vi "SelectBeads.vi"(11 "Input image":T1) -> ()   [LabVIEW 2011]
uses:
  <vilib>/vision/Image Controls.llb/IMAQ Image.ctl
  GlobalVariables.vi
panel:
  in  "Use old?":bool
  in  "error in (no error)":errorcluster
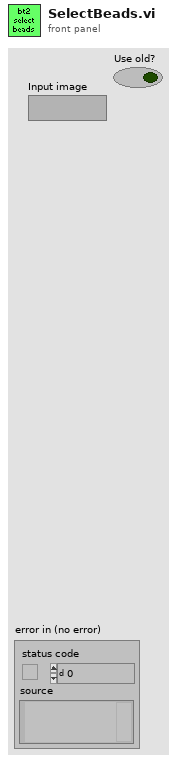
[diagram p1: front panel]
types:
  T1 = typedef "IMAQ Image.ctl" = refnum<image>
  T2 = typedef "MeasureConfigType.ctl" = cluster{"Bead locations":cluster{"X":i32, "Y":i32}[], "ROI":i32, "Experiment base path":path, "Image output subdir":string, "Output mode":T3, "Traces output subdir":string, "QTrk Settings":T4, "Tracking Config":T5, "Experiment Name":string, "Program":T8, "ZLUT":sgl[][][], "Camera settings":T15, "Experiment Script":string, "Max frames in memory":i32, "Save traces as binary":bool, "Pixel Calibration Gain Image":string, "Pixel Calibration Offset Image":string, "Use pixel calibration images":bool, "Internal camera settings":string}
  T3 = typedef "MeasureConfigOutputMode.ctl" = enum16{"None", "Track", "SaveImages"}
  T4 = typedef "QTrkSettings.ctl" = cluster{"Image width":i32, "Image height":i32, "Number of threads (CPU based)":i32, "CUDA Device":i32, "COM Background correction factor":sgl, "ZLUT MinRadius":sgl, "ZLUT Radial sample density":sgl, "ZLUT Angular sample density":sgl, "ZLUT ROI Coverage":sgl, "QI Iterations":i32, "QI MinRadius":sgl, "QI Radial sample density":sgl, "QI Angular sample density":sgl, "QI ROI Coverage":sgl, "QI Angular Step \nIteration Factor":sgl, "XCOR Profile Length":i32, "XCOR Profile Width":i32, "XCOR Iterations":i32, "Gaussian 2D Fit Iterations":i32, "Gaussian 2D Sigma (pixels)":sgl}
  T5 = typedef "TrackingConfigType.ctl" = cluster{"Number of steps":i32, "ZLUT stepsize (um)":sgl, "Z correction factor":sgl, "Start piezo Z (um)":sgl, "Pixel size (nm)":sgl, "2D Localization Type":T6, "Z Command (None)":T7, "Z Piezo scale":bool}
  T6 = typedef "QTrkLocalizationType.ctl" = enum16{"Center-of-Mass", "1D Cross-Correlation", "Quadrant Interpolation", "Gaussian 2D MLE", "QI + ZLUTAlign", "ZLUTAlign"}
  T7 = typedef "QTrkZCommandType.ctl" = enum16{"Nothing", "ComputeZ", "BuildRadialZLUT", "BuildImageZLUT", "RadialZLUT+ImageZLUT"}
  T8 = typedef "ExperimentProgramType.ctl" = cluster{"Commands":T9[], "Motor Axis accuracy conditions":T12, "Axis flags":T14}
  T9 = typedef "ExProgCommandType.ctl" = cluster{"cmd":T10, "axis":T11, "value/pos":dbl, "speed":dbl, "name":string}
  T10 = typedef "ExProgCommandEnumType.ctl" = enum16{"wait", "move", "acquire", "idle", "rmove", "when", "section", "stop"}
  T11 = typedef "MotorAxisEnum.ctl" = enum16{"no axis", "magrot", "magpos", "px", "py", "pz", "camx", "camy"}
  T12 = typedef "MotorPosType.ctl" = cluster{"Magnet Z":dbl, "Magnet rotation":dbl, "Camera":T13, "Piezo XY":T13, "Piezo Z":dbl}
  T13 = typedef "XYf.ctl" = cluster{"X":sgl, "Y":sgl}
  T14 = typedef "MotorPosFlagsType.ctl" = cluster{"Magnet Z":bool, "Magnet rotation":bool, "Camera":cluster{"X":bool, "Y":bool}, "Piezo XY":cluster{"X":bool, "Y":bool}, "Piezo Z":bool}
  T15 = typedef "GenericCameraConfigType.ctl" = cluster{"Framerate (Hz)":i32, "Exposure time (us)":i32, "Image size":cluster{"Width":i32, "Height":i32}, "Number of buffers":i32}
  T16 = typedef "CameraInstance.ctl" = cluster{"VI refs":T17, "Camera state":variant}
  T17 = typedef "CameraInterface.ctl" = cluster{"Close":T18, "Get/Set generic config":T19, "Grab":T20, "Show Settings Dialog":T21, "AdjustBeadPos":T22, "Save/load camera settings":T23}
  T18 = typedef "CICloseType.ctl" = refnum<vi>
  T19 = typedef "CIGetSetGenericConfig.ctl" = refnum<vi>
  T20 = typedef "CIGrabType.ctl" = refnum<vi>
  T21 = typedef "CISettingsDlg.ctl" = refnum<vi>
  T22 = typedef "CIAdjustBeadPos.ctl" = refnum<vi>
  T23 = typedef "CISaveLoadSettings.ctl" = refnum<vi>
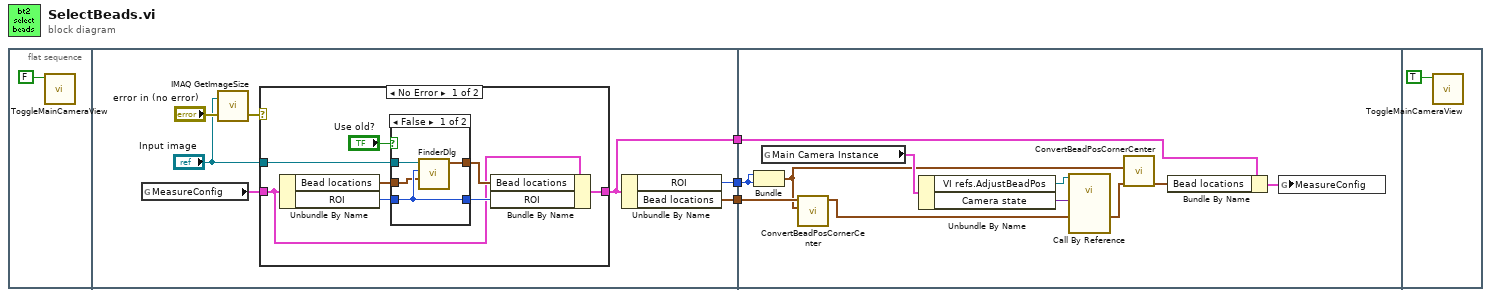
[diagram p0: block diagram]
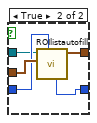
[diagram p2: hidden frame]
diagram:
  n1 = flat-sequence {
    tunnel: [w7] -> w3
    tunnel: [w6] -> w2
    tunnel: [w5] -> w1
    tunnel: w3 -> [w35]
    tunnel: w2 -> [w38]
    tunnel: w1 -> [w34]
    frame #0 {
      n2 = call "ToggleMainCameraView.vi"("Enable? (T)"=FALSE) -> ()  [unwired: 11 in]
    }
    frame #1 {
      n3 = global read "GlobalVariables.vi" "MeasureConfig"() -> (w8:T2)
      n4 = call "IMAQ GetImageSize"("Image"="Input image", "error in (no error)"="error in (no error)") -> ("error out"=w11:errorcluster)  [unwired: 2 in, 2 out]
      n5 = case shown="No Error" w11 {
        tunnel: "Input image" -> [w15 _]
        tunnel: w8 -> [w14 w29]
        tunnel: [w13 w29] -> w6
        frame No Error {
          n6 = Unbundle By Name(w14) -> ("Bead locations"=w19:cluster{"X":i32, "Y":i32}[], "ROI"=w18:i32)
          n7 = case shown="False" "Use old?" {
            tunnel: w19 -> [w20 w28]
            tunnel: w18 -> [w22 w27]
            tunnel: [w21 w26] -> w17
            tunnel: [w22 w25] -> w16
            tunnel: w15 -> [w23 w24]
            frame False {
              n8 = call "FinderDlg.vi"("Bead positions"=w20, "roi"=w22, "Input Image"=w23) -> ("Bead positions"=w21:cluster{"X":i32, "Y":i32}[])  [unwired: 8 in]
            }
            frame True {
              n9 = call "ROIlistautofill.vi"("ROI in (pix)"=w27, "Bead locations"=w28, "Image In"=w24) -> ("Output bead locations"=w26:cluster{"X":i32, "Y":i32}[], "ROI out"=w25:i32)  [unwired: 4 in, 3 out]
            }
          }
          n10 = Bundle By Name(cluster=w14, "Bead locations"=w17, "ROI"=w16) -> (w13:T2)
        }
        frame Error {
        }
      }
      n11 = Unbundle By Name(w6) -> ("ROI"=w5:i32, "Bead locations"=w7:cluster{"X":i32, "Y":i32}[])
    }
    frame #2 {
      n12 = Bundle("ROI"=w34, "ROI"=w34) -> (w32:cluster{"ROI":i32, "ROI":i32})  [unwired: 1 in]
      n13 = global read "GlobalVariables.vi" "Main Camera Instance"() -> (w36:T16)
      n14 = call "ConvertBeadPosCornerCenter.vi"("ROI Size"=w32, "Center-based bead locations"=w35) -> ("Corner-based bead pos (out)"=w33:cluster{"X":i32, "Y":i32}[])  [unwired: 8 in, 1 out]
      n15 = Unbundle By Name(w36) -> ("VI refs.AdjustBeadPos"=w39:T22, "Camera state"=w40:variant)
      n16 = call-by-ref "?"(reference=w39, "Corner-based bead pos"=w33, "Camera state"=w40) -> ("Adjusted bead pos (out)"=w31:cluster{"X":i32, "Y":i32}[])  [unwired: 9 in, 3 out]
      n17 = call "ConvertBeadPosCornerCenter.vi"("Corner-based bead locations"=w31, "ROI Size"=w32) -> ("Center-based bead pos (out)"=w30:cluster{"X":i32, "Y":i32}[])  [unwired: 8 in, 1 out]
      n18 = Bundle By Name(cluster=w38, "Bead locations"=w30) -> (w37:T2)
      n19 = global write "GlobalVariables.vi" "MeasureConfig"(w37) -> ()
    }
    frame #3 {
      n20 = call "ToggleMainCameraView.vi"("Enable? (T)"=TRUE) -> ()  [unwired: 11 in]
    }
  }
